vi "Hybrid PS Set Pause.vi"(0 "Pause":bool, 1 "Change it":bool, 2 "VI Refnum":refnum<vi>) -> ()   [LabVIEW 2021]
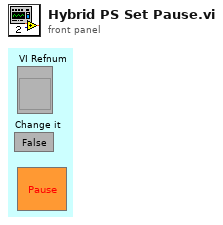
[diagram p1: front panel]
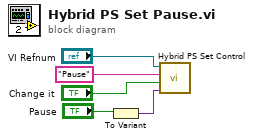
[diagram p0: block diagram]
diagram:
  n1 = To Variant(anything="Pause") -> (Variant=w5:variant)
  n2 = call "Hybrid PS Set Control.vi"("Value"=w5, "Change it"="Change it", "Control Name"="Pause", "VI Refnum"="VI Refnum") -> ()
